vi "GenNet Send Message.vi"(6 "timeout [ms]":i32=100, 8 "error in (no error)":errorcluster, 10 "Message Data":variant, 11 "TCP Network Connection in":refnum<k5>) -> (0 "error out":errorcluster, 3 "TCP Network Connection out":refnum<k5>)   [LabVIEW 2014, in "hse-gennet.lvlib"]
doc: "Sends a message via TCP/IP to a GenNet-Server module. \n\nThe message is flattened to a string, and the length of the string is prepended before sending it over the network.\n\n____\nHAMPEL SOFTWARE ENGINEERING v0.7.0 (2018-07-16 18:12)"
uses:
  hse-gennet.lvlib
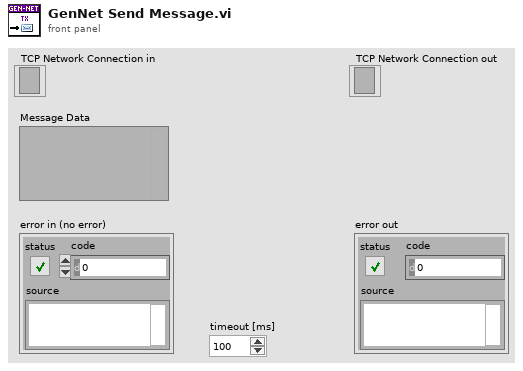
[diagram p1: front panel]
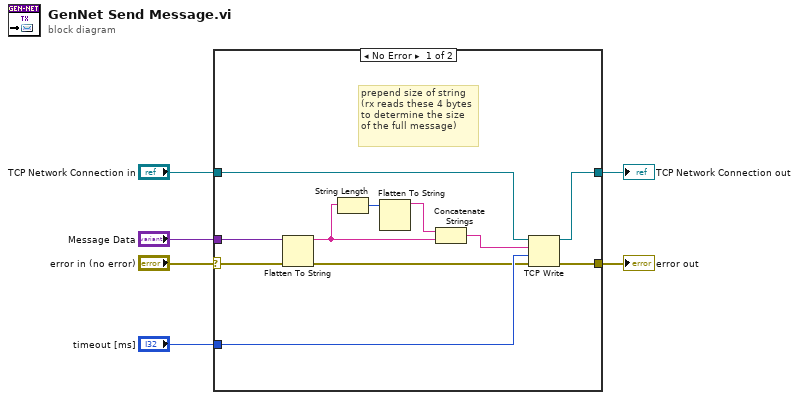
[diagram p0: block diagram]
diagram:
  n1 = case shown="No Error" "error in (no error)" {
    selector: "error in (no error)" -> [w10 w18]
    tunnel: "TCP Network Connection in" -> [w17 w19]
    tunnel: [w13 w18] -> w5
    tunnel: [w12 w19] -> w4
    tunnel: "Message Data" -> [w8 _]
    tunnel: "timeout [ms]" -> [w11 _]
    frame No Error {
      # "prepend size of string\n(rx reads these 4 bytes\nto determine the size\nof the full message)"
      n2 = Flatten To String(anything=w8, error in (no error)=w10) -> (data string=w7:string, error out=w9:errorcluster)  [unwired: 2 in, 1 out]
      n3 = String Length(string=w7) -> (length=w14:i32)
      n4 = Flatten To String(anything=w14) -> (data string=w15:string)  [unwired: 3 in, 2 out]
      n5 = Concatenate Strings(w15, w7) -> (w16:string)
      n6 = TCP Write(connection ID=w17, data in=w16, error in (no error)=w9, 9:w11) -> (connection ID out=w12:refnum<k5>, error out=w13:errorcluster)  [unwired: 1 out]
    }
    frame Error {
    }
  }
  "error out" <- w5
  "TCP Network Connection out" <- w4
